vi "execute.vi"(8 "error in (no error)":errorcluster, 9 "data collection in":refnum<class "GenericComponent.lvclass">, 10 "imaging mode  in":refnum<class "GenericComponent.lvclass">, 11 "adapter in":refnum<class "AdapterMG091111ImagingModeToDataCollection.lvclass">) -> (0 "error out":errorcluster, 1 "data collection out":refnum<class "GenericComponent.lvclass">, 2 "imaging mode out":refnum<class "GenericComponent.lvclass">, 3 "adapter out":refnum<class "AdapterMG091111ImagingModeToDataCollection.lvclass">)   [LabVIEW 2010, in "AdapterMG091111ImagingModeToDataCollection.lvclass"]
uses:
  AdapterMG091111ImagingModeToDataCollection.lvclass
  common/classes/GenericComponent/GenericComponent/GenericComponent.lvclass
  ImagingMode/ImagingModeMG091111IntrinsicImaging/ImagingModeMG091111IntrinsicImaging/ImagingModeMG091111IntrinsicImaging.lvclass
  DataCollection/DataCollectionMG091001IntrinsicImaging/DataCollectionMG091001IntrinsicImaging/DataCollectionMG091001IntrinsicImaging.lvclass
panel:
  # "imaging mode: ImagingModeMG091111IntrinsicImaging\ndata collection: DataCollectionMG091001IntrinsicImaging"
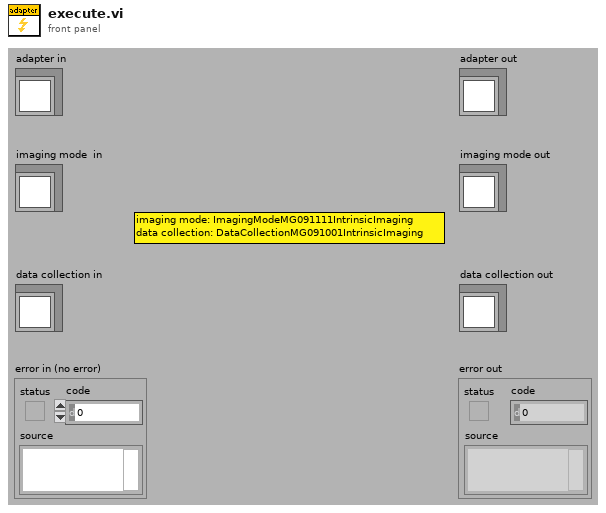
[diagram p1: front panel]
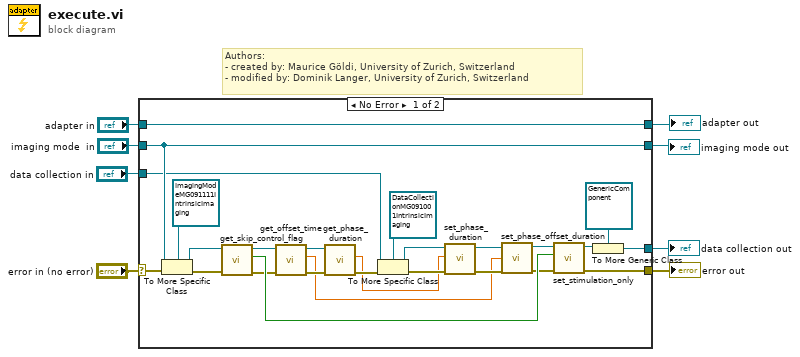
[diagram p0: block diagram]
diagram:
  # "Authors: \n- created by: Maurice Göldi, University of Zurich, Switzerland\n- modified by: Dominik Langer, University of Zurich, Switzerland"
  n1 = case shown="No Error" "error in (no error)" {
    selector: "error in (no error)" -> [w33 w37]
    tunnel: [w34 w38] -> w7
    tunnel: "adapter in" -> [w34 w38]
    tunnel: [w19 w37] -> w5
    tunnel: "imaging mode  in" -> [w32 w36]
    tunnel: [w32 w36] -> w3
    tunnel: [w26 w35] -> w2
    tunnel: "data collection in" -> [w31 w35]
    frame No Error {
      n2 = To More Specific Class(target class=refnum<class "ImagingModeMG091111IntrinsicImaging.lvclass"> refnum ("ImagingModeMG091111IntrinsicImaging.lvclass"), reference=w32, error in=w33) -> (specific class reference=w21:refnum<class "ImagingModeMG091111IntrinsicImaging.lvclass">, error out=w22:errorcluster)
      n3 = call-dynamic "get_skip_control_flag.vi"("error in (no error)"=w22, "ScanModeMG091111IntrinsicImaging in"=w21) -> ("error out"=w12:errorcluster, "skip control?"=w13:bool, "ScanModeMG091111IntrinsicImaging out"=w11:refnum<class "ImagingModeMG091111IntrinsicImaging.lvclass">)  [unwired: 7 in]
      n4 = call-dynamic "get_offset_time.vi"("error in (no error)"=w12, "ScanModeMG091111IntrinsicImaging in"=w11) -> ("error out"=w24:errorcluster, "offset time"=w15:dbl[unit], "ScanModeMG091111IntrinsicImaging out"=w23:refnum<class "ImagingModeMG091111IntrinsicImaging.lvclass">)  [unwired: 7 in]
      n5 = call-dynamic "get_phase_duration.vi"("error in (no error)"=w24, "ScanModeMG091111IntrinsicImaging in"=w23) -> ("error out"=w25:errorcluster, "phase duration"=w14:dbl[unit])  [unwired: 7 in, 1 out]
      n6 = To More Specific Class(target class=refnum<class "DataCollectionMG091001IntrinsicImaging.lvclass"> refnum ("DataCollectionMG091001IntrinsicImaging.lvclass"), reference=w31, error in=w25) -> (specific class reference=w16:refnum<class "DataCollectionMG091001IntrinsicImaging.lvclass">, error out=w17:errorcluster)
      n7 = call "set_phase_duration.vi"("error in (no error)"=w17, "phase duration"=w14, "IntrinsicImagingMG091001 in"=w16) -> ("error out"=w28:errorcluster, "IntrinsicImagingMG091001 out"=w27:refnum<class "DataCollectionMG091001IntrinsicImaging.lvclass">)  [unwired: 7 in]
      n8 = call "set_phase_offset_duration.vi"("error in (no error)"=w28, "phase offset duration"=w15, "IntrinsicImagingMG091001 in"=w27) -> ("error out"=w10:errorcluster, "IntrinsicImagingMG091001 out"=w9:refnum<class "DataCollectionMG091001IntrinsicImaging.lvclass">)  [unwired: 7 in]
      n9 = call-dynamic "set_stimulation_only.vi"("error in (no error)"=w10, "stimulation only?"=w13, "IntrinsicImagingMG091001 in"=w9) -> ("error out"=w19:errorcluster, "IntrinsicImagingMG091001 out"=w18:refnum<class "DataCollectionMG091001IntrinsicImaging.lvclass">)  [unwired: 7 in]
      n10 = To More Generic Class(target class=refnum<class "GenericComponent.lvclass"> refnum ("GenericComponent.lvclass"), reference=w18) -> (generic class reference=w26:refnum<class "GenericComponent.lvclass">)
    }
    frame Error {
    }
  }
  "error out" <- w5
  "adapter out" <- w7
  "imaging mode out" <- w3
  "data collection out" <- w2
